vi "AutoHelper_Sequence_Execute.vi"(4 "Set Next Step":bool, 6 "Pass_Through_Time":dbl=-1.0 format="%33.4f", 8 "Use Custom Next Step":bool, 9 "Custom Step Number":T1=enum."Step 1", 10 "Initiate":bool, 11 "Step Times Sec":dbl[](array[numeric])) -> (0 "Error":bool, 1 "Elapsed Step Time":dbl, 2 "Seq  Active":bool, 3 "Step Number State":T1, 5 "New Step":bool)   [LabVIEW 2019, in "Trajectory_Library.lvlib"]
doc: "Implements a simplified state machine similar to a mechanical / electrical drum sequencer. When the Drum Sequencer is \"Ready\" and the \"Initiate\" input becomes TRUE,, the drum sequences through its set of steps from 1 to N. After each Step is executed it is followed by a wait. During the wait the Step output indicates \"Do Nothing\". The number of Steps is determined by the number of elements in the \"Step Times\" input array. Once all the steps have been executed, the Drum Sequencer cycles bac to wait for another initiate. \n\nThere is a Cancel input that interrupts the sequence, executes the Cancel Step, performs the cancel wait, and then returns to wait for an Initiate action. \n\nIf any of the Step Times, or Cancel times are negative, or there more than 32 steps, or less than 1 step an error is signaled. The drum sequencer selects the error state and stays there.\n\nInputs:\n\nOutputs:"
uses:
  Trajectory_Library.lvlib
  Enum/AutoHelperSequence_Step_Enum.ctl
  Enum/DrumSequence_State_Enum.ctl
  Util_GetTime_U32.vi
  Util_GetTime_U64.vi
  <vilib>/Utility/semaphor.llb/Obtain Semaphore Reference.vi
  Timer_Reset.vi
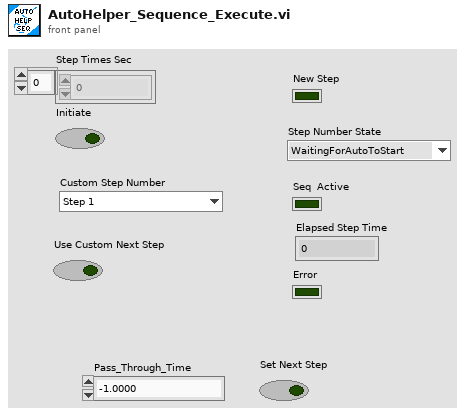
[diagram p1: front panel]
types:
  T1 = typedef "Trajectory_Library.lvlib/AutoHelperSequence_Step_Enum.ctl" = enum16{"WaitingForAutoToStart", "Step 1", "Step 2", "Step 3", "Step 4", "Step 5", "Step 6", "Step 7", "Step 8", "Step 9", "Step 10", "Step 11", "Step 12", "Step 13", "Step 14", "Step 15", "Step 16", "Step 17", "Step 18", "Step 19", "Step 20", "Step 21", "Step 22", "Step 23", "Step 24", "Step 25", "Step 26", "Step 27", "Step 28", "Step 29", "Step 30", "Step 31", "Step 32", "AutoDone"}
  T2 = typedef "Trajectory_Library.lvlib/DrumSequence_State_Enum.ctl" = enum16{"Initialize", "Ready", "First Step", "Step Wait", "Next State", "Cancel", "Cancel Wait", "Error", "Error Loop"}
  T3 = typedef "Trajectory_Library.lvlib/TIMER.ctl" = cluster{"StartTime":dbl, "Accumulated TIme":dbl, "Running":bool, "semaphore":T4}
  T4 = typedef "Semaphore RefNum" = refnum<k1>
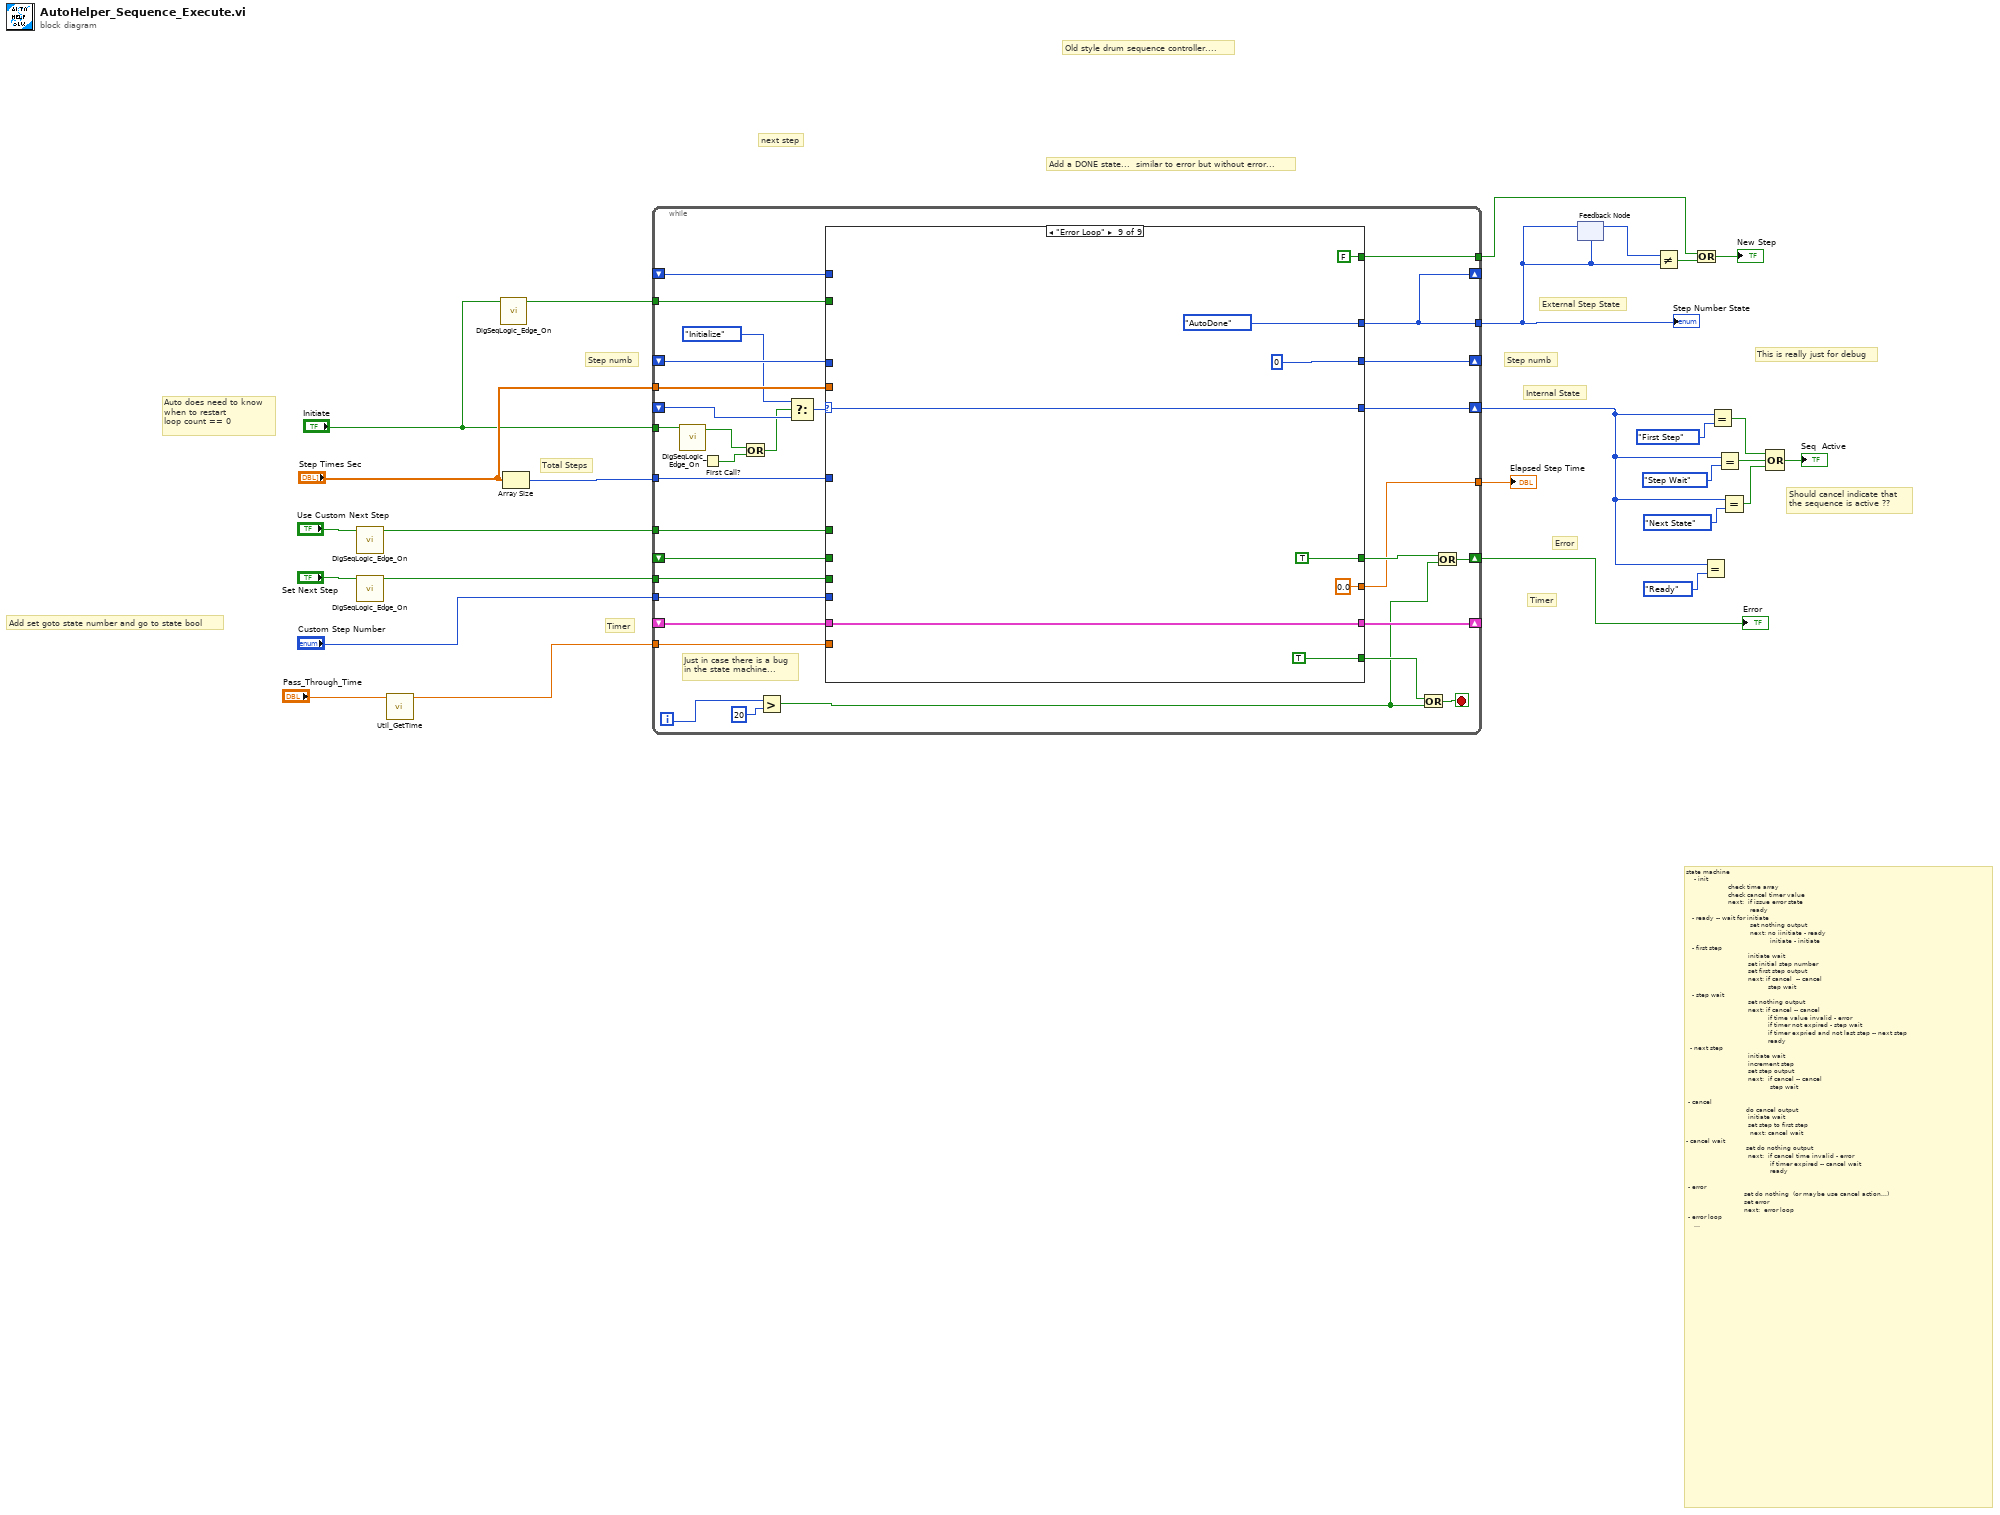
[diagram p0: block diagram]
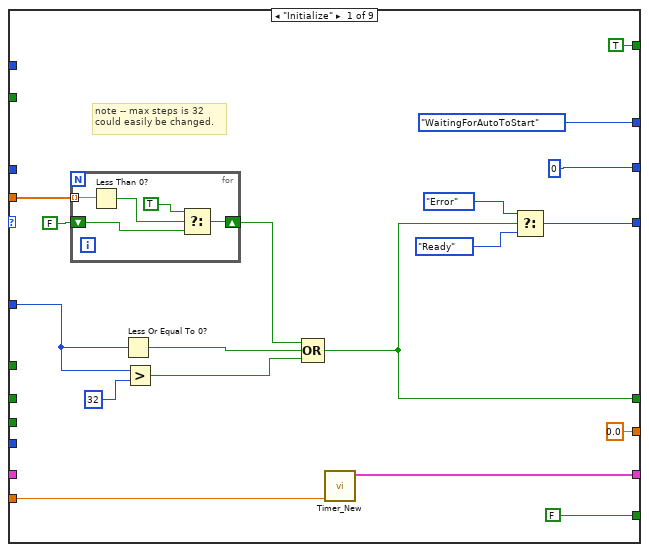
[diagram p2: hidden frame]
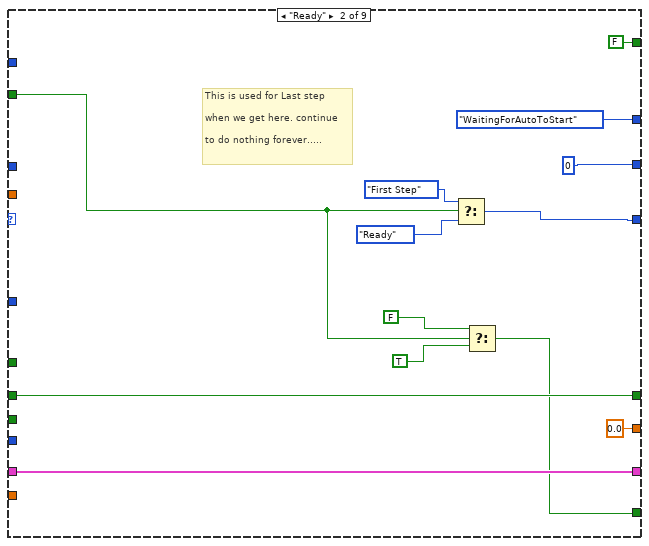
[diagram p3: hidden frame]
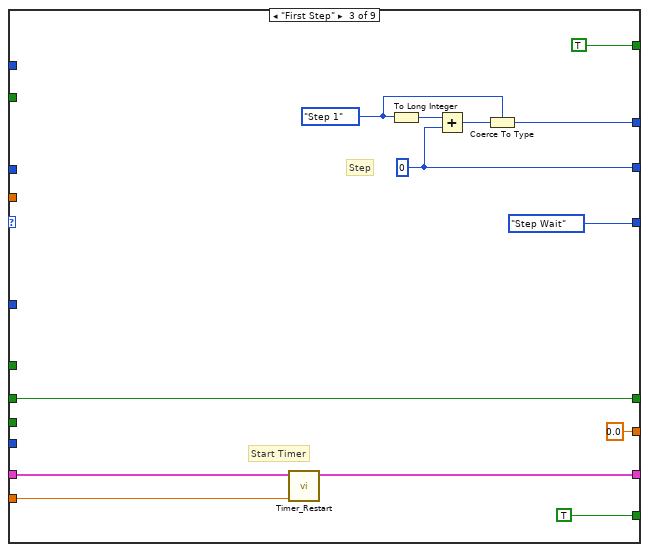
[diagram p4: hidden frame]
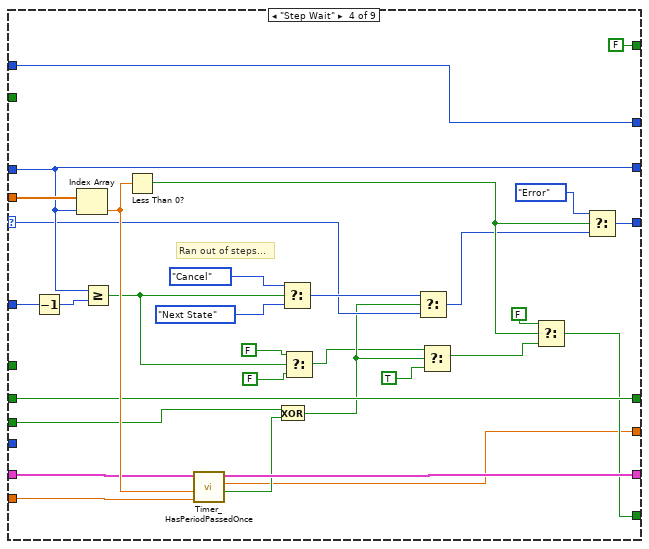
[diagram p5: hidden frame]
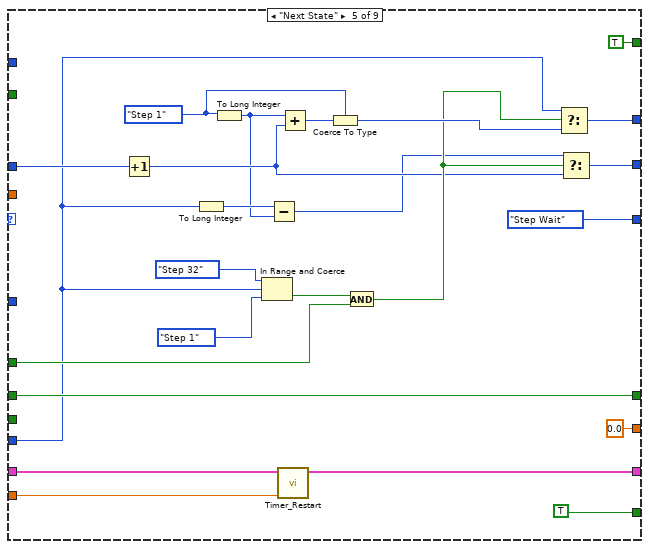
[diagram p6: hidden frame]
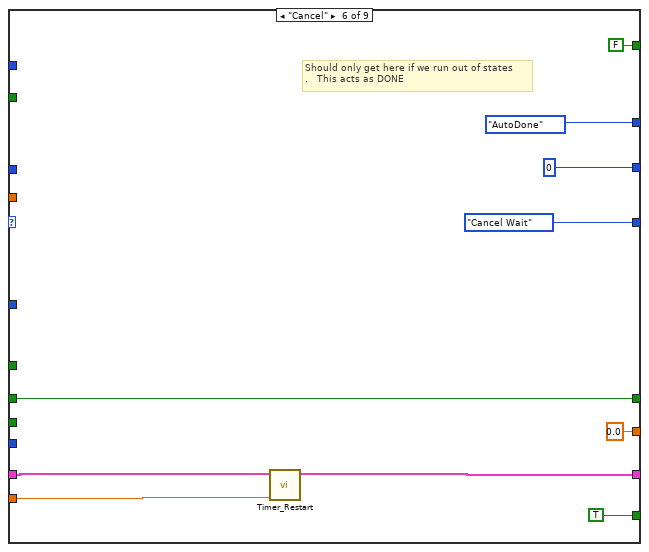
[diagram p7: hidden frame]
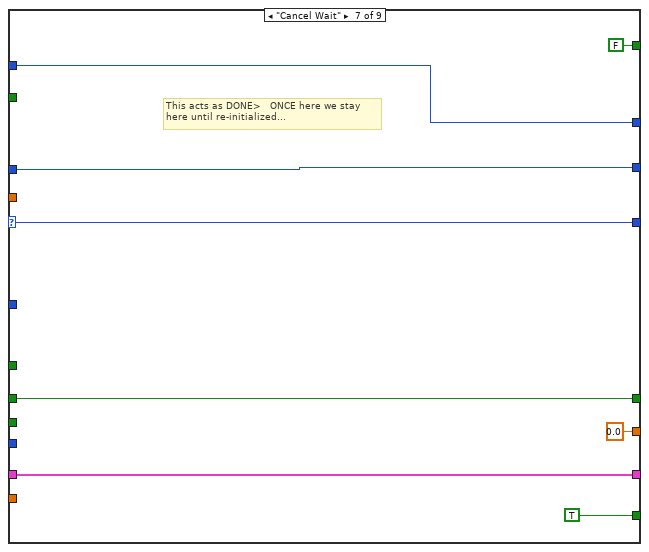
[diagram p8: hidden frame]
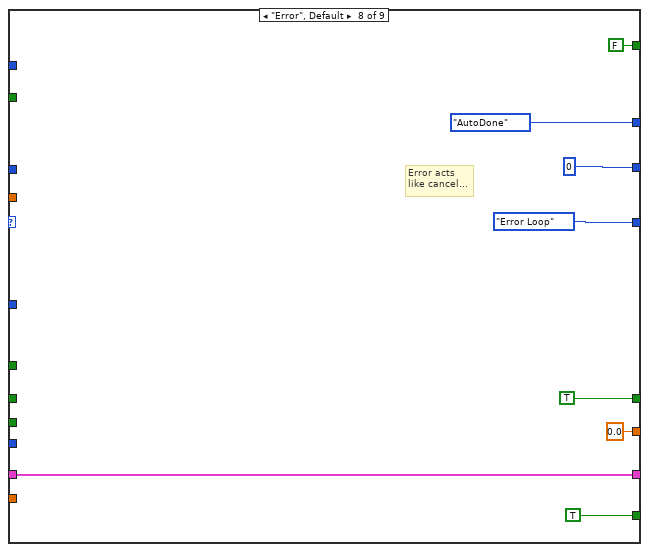
[diagram p9: hidden frame]
diagram:
  # "Add a DONE state...  similar to error but without error..."
  # "Add set goto state number and go to state bool"
  # "Auto does need to know\nwhen to restart\nloop count == 0"
  # "Should cancel indicate that\nthe sequence is active ??"
  # "This is really just for debug"
  # "Timer"
  # "Total Steps"
  # "Step numb"
  # "next step"
  # "Old style drum sequence controller...."
  # "Step numb"
  # "Timer"
  # "Error"
  # "Internal State"
  # "External Step State"
  # "state machine\n    - init\n                     check time array\n                     check cancel timer value\n                     next:  if issue error state\n                                ready\n   - ready -- wait for initiate\n                                set nothing output\n                                next: no iinitiate - ready\n                                          initiate - initiate\n   - first step \n                               initiate wait\n                               set initial step number\n                               set first step output\n                               next: if cancel  -- cancel\n                                         step wait\n   - step wait \n                               set nothing output\n                               next: if cancel -- cancel\n                                         if time value invalid - error\n                                         if timer not expired - step wait\n                                         if timer expried and not last step -- next step\n                                         ready\n  - next step\n                               initiate wait\n                               increment step\n                               set step output\n                               next:  if cancel -- cancel\n                                          step wait\n\n - cancel\n                              do cancel output\n                               initiate wait\n                               set step to first step\n                                next: cancel wait\n- cancel wait\n                              set do nothing output\n                               next:  if cancel time invalid - error\n                                          if timer expired -- cancel wait\n                                          ready\n\n - error\n                             set do nothing  (or maybe use cancel action...)\n                             set error\n                             next:  error loop\n - error loop\n                             set do nothing\n                             set error\n                             next: error loop"
  n1 = call "DigSeqLogic_Edge_On.vi"("Input"="Use Custom Next Step") -> ("On Edge"=w4:bool)  [unwired: 10 in]
  n2 = call "DigSeqLogic_Edge_On.vi"("Input"="Set Next Step") -> ("On Edge"=w13:bool)  [unwired: 10 in]
  n3 = call "Util_GetTime.vi"("Pass_Through_Time"="Pass_Through_Time") -> ("FPGA_Time_Seconds"=w24:dbl)  [unwired: 8 in, 2 out]
  n4 = call "DigSeqLogic_Edge_On.vi"("Input"="Initiate") -> ("On Edge"=w1:bool)  [unwired: 10 in]
  n5 = Array Size(array="Step Times Sec") -> (size(s)=w27:i32)
  n6 = while {
    tunnel: "Step Times Sec" -> [w57]
    tunnel: w24 -> [w56]
    tunnel: [w38] -> w8
    tunnel: w13 -> [w53]
    tunnel: w27 -> [w58]
    shift-right: [w52] -> _
    shift-left: _ -> [w46]
    shift-right: [w41] -> w12
    shift-left: _ -> [w51]
    shift-right: [w54] -> w15
    shift-left: _ -> [w48]
    shift-right: [w55] -> _
    shift-left: _ -> [w50]
    shift-right: [w38] -> _
    shift-left: _ -> [w37]
    tunnel: "Initiate" -> [w29]
    tunnel: [w34] -> w7
    tunnel: [w33] -> w6
    tunnel: w4 -> [w32]
    tunnel: "Custom Step Number" -> [w31]
    tunnel: w1 -> [w28]
    i -> [w43]
    stop <- w45 stop-if-true
    # "Just in case there is a bug\nin the state machine..."
    n7 = call "DigSeqLogic_Edge_On.vi"("Input"=w29) -> ("On Edge"=w30:bool)  [unwired: 10 in]
    n8 = First Call?() -> (First Call?: T/F=w36:bool)
    n9 = Or(x=w30, y=w36) -> (x .or. y?=w35:bool)
    n10 = Greater?(x=w43, y=20) -> (0:w39:bool)
    n11 = Select(t=DrumSequence_State_Enum."Initialize", s=w35, f=w48) -> (s? t:f=w49:T2)
    n12 = case shown="\"Error Loop\"" w49 {
      selector: w49 -> [_ _ _ w128 _ _ w174 _ w195]
      tunnel: w58 -> [w66 _ _ w126 _ _ _ _ _]
      tunnel: w57 -> [w75 _ _ w133 _ _ _ _ _]
      tunnel: [w72 w92 w99 w122 w157 w167 w179 TRUE TRUE] -> w40
      tunnel: [w69 w83 DrumSequence_State_Enum."Step Wait" w130 DrumSequence_State_Enum."Step Wait" DrumSequence_State_Enum."Cancel Wait" w174 DrumSequence_State_Enum."Error Loop" w195] -> w54
      tunnel: [w68 w91 w102 w137 w159 w170 w176 w183 w192] -> w52
      tunnel: w56 -> [w67 _ w103 w138 w160 w171 _ _ _]
      tunnel: [AutoHelperSequence_Step_Enum."WaitingForAutoToStart" ("Auto Helper Step Number") AutoHelperSequence_Step_Enum."WaitingForAutoToStart" ("Auto Helper Step Number") w105 w112 w147 AutoHelperSequence_Step_Enum."AutoDone" ("Auto Helper Step Number") w178 AutoHelperSequence_Step_Enum."AutoDone" ("Auto Helper Step Number") AutoHelperSequence_Step_Enum."AutoDone" ("Auto Helper Step Number")] -> w38
      tunnel: [0 0 w104 w129 w145 0 w180 0 0] -> w55
      tunnel: w50 -> [_ _ _ w129 w161 _ w180 _ _]
      tunnel: w53 -> [_ _ _ w124 _ _ _ _ _]
      tunnel: w46 -> [_ w91 w100 w123 w156 w165 w176 w183 w192]
      tunnel: w51 -> [_ w92 w99 w122 w157 w167 w179 _ _]
      tunnel: [FALSE w84 TRUE w113 TRUE TRUE TRUE TRUE TRUE] -> w44
      tunnel: w37 -> [_ _ _ w112 _ _ w178 _ _]
      tunnel: [TRUE FALSE TRUE FALSE TRUE FALSE FALSE FALSE FALSE] -> w34
      tunnel: [0.0 ("CurrentTImer") 0.0 ("CurrentTImer") 0.0 ("CurrentTImer") w108 0.0 ("CurrentTImer") 0.0 ("CurrentTImer") 0.0 ("CurrentTImer") 0.0 ("CurrentTImer") 0.0 ("CurrentTImer")] -> w33
      tunnel: w32 -> [_ _ _ _ w148 _ _ _ _]
      tunnel: w31 -> [_ _ _ _ w142 _ _ _ _]
      tunnel: w28 -> [_ w82 _ _ _ _ _ _ _]
      frame "Initialize" {
        # "note -- max steps is 32\ncould easily be changed."
        n13 = for {
          shift-right: [w80] -> w74
          shift-left: FALSE -> [w79]
          tunnel: w75 -> [w81] mode=indexing
          n14 = Less Than 0?(x=w81) -> (x < 0?=w77:bool)
          n15 = Select(t=TRUE, s=w77, f=w79) -> (s? t:f=w80:bool)
        }
        n16 = Less Or Equal To 0?(x=w66) -> (x <= 0?=w73:bool)
        n17 = Greater?(x=w66, y=32) -> (0:w61:bool)
        n18 = Compound Arithmetic op=OR(w74, w73, w61) -> (w72:bool)
        n19 = call "Timer_New.vi"("Pass_Through_Time"=w67) -> ("TIMER"=w68:T3)  [unwired: 10 in]
        n20 = Select(t=DrumSequence_State_Enum."Error", s=w72, f=DrumSequence_State_Enum."Ready") -> (s? t:f=w69:T2)
      }
      frame "Ready" {
        # "This is used for Last step\n\nwhen we get here. continue\n\nto do nothing forever....."
        n21 = Select(t=DrumSequence_State_Enum."First Step", s=w82, f=DrumSequence_State_Enum."Ready") -> (s? t:f=w83:T2)
        n22 = Select(t=FALSE, s=w82, f=TRUE) -> (s? t:f=w84:bool)
      }
      frame "First Step" {
        w101 = AutoHelperSequence_Step_Enum."Step 1" ("Auto Helper Step Number")
        w104 = 0
        # "Start Timer"
        # "Step"
        n23 = call "Timer_Restart.vi"("Pass_Through_Time"=w103, "in Timer"=w100) -> ("out Timer"=w102:T3)  [unwired: 9 in]
        n24 = To Long Integer(number=w101) -> (32bit integer=w107:i32)
        n25 = Add(x=w107, y=w104) -> (x+y=w106:i32)
        n26 = Coerce To Type(0:w106, 1:w101) -> (2:w105:T1)
      }
      frame "Step Wait" {
        # "Ran out of steps..."
        n27 = Decrement(x=w126) -> (x-1=w127:i32)
        n28 = Index Array(array=w133, index=w129) -> (element=w132:dbl)
        n29 = Greater Or Equal?(x=w129, y=w127) -> (x >= y?=w121:bool)
        n30 = Less Than 0?(x=w132) -> (x < 0?=w114:bool)
        n31 = call "Timer_HasPeriodPassedOnce.vi"("Pass_Through_Time"=w138, "Period"=w132, "in Timer"=w123) -> ("Expired"=w125:bool, "CurrentTImer"=w108:dbl, "out Timer"=w137:T3)  [unwired: 6 in]
        n32 = Exclusive Or(1:w125, 2:w124) -> (0:w118:bool)
        n33 = Select(t=DrumSequence_State_Enum."Cancel", s=w121, f=DrumSequence_State_Enum."Next State") -> (s? t:f=w134:T2)
        n34 = Select(t=FALSE, s=w121, f=FALSE) -> (s? t:f=w117:bool)
        n35 = Select(t=w134, s=w118, f=w128) -> (s? t:f=w111:T2)
        n36 = Select(t=w117, s=w118, f=TRUE) -> (s? t:f=w110:bool)
        n37 = Select(t=FALSE, s=w114, f=w110) -> (s? t:f=w113:bool)
        n38 = Select(t=DrumSequence_State_Enum."Error", s=w114, f=w111) -> (s? t:f=w130:T2)
      }
      frame "Next State" {
        w158 = AutoHelperSequence_Step_Enum."Step 1" ("Auto Helper Step Number")
        n39 = Increment(x=w161) -> (x+1=w143:i32)
        n40 = To Long Integer(number=w142) -> (32bit integer=w141:i32)
        n41 = To Long Integer(number=w158) -> (32bit integer=w140:i32)
        n42 = In Range and Coerce(upper limit=AutoHelperSequence_Step_Enum."Step 32" ("Auto Helper Step Number"), x=w142, lower limit=AutoHelperSequence_Step_Enum."Step 1" ("Auto Helper Step Number")) -> (In Range?=w149:bool)  [unwired: 1 out]
        n43 = Subtract(x=w141, y=w140) -> (x-y=w139:i32)
        n44 = call "Timer_Restart.vi"("Pass_Through_Time"=w160, "in Timer"=w156) -> ("out Timer"=w159:T3)  [unwired: 9 in]
        n45 = Add(x=w140, y=w143) -> (x+y=w162:i32)
        n46 = Coerce To Type(0:w162, 1:w158) -> (2:w146:T1)
        n47 = And(x=w149, y=w148) -> (x .and. y?=w144:bool)
        n48 = Select(t=w142, s=w144, f=w146) -> (s? t:f=w147:T1)
        n49 = Select(t=w139, s=w144, f=w143) -> (s? t:f=w145:i32)
      }
      frame "Cancel" {
        # "Should only get here if we run out of states\n.   This acts as DONE"
        n50 = call "Timer_Restart.vi"("Pass_Through_Time"=w171, "in Timer"=w165) -> ("out Timer"=w170:T3)  [unwired: 9 in]
      }
      frame "Cancel Wait" {
        # "This acts as DONE>   ONCE here we stay \nhere until re-initialized..."
      }
      frame "Error", Default {
        # "Error acts\nlike cancel..."
      }
      frame "Error Loop" {
      }
    }
    n51 = Or(x=w44, y=w39) -> (x .or. y?=w45:bool)
    n52 = Or(x=w40, y=w39) -> (x .or. y?=w41:bool)
  }
  "Error" <- w12
  "Step Number State" <- w8
  "Elapsed Step Time" <- w6
  n53 = feedback #1(w8) -> (w11:T1)
  n54 = feedback-in #1(w8) -> ()
  n55 = Not Equal?(x=w11, y=w8) -> (x != y?=w9:bool)
  n56 = Or(x=w7, y=w9) -> (x .or. y?=→"New Step":bool)
  n57 = Equal?(x=w15, y=DrumSequence_State_Enum."Ready") -> ()  [unwired: 1 out]
  n58 = Equal?(x=w15, y=DrumSequence_State_Enum."First Step") -> (x = y?=w19:bool)
  n59 = Equal?(x=w15, y=DrumSequence_State_Enum."Step Wait") -> (x = y?=w18:bool)
  n60 = Equal?(x=w15, y=DrumSequence_State_Enum."Next State") -> (x = y?=w17:bool)
  n61 = Compound Arithmetic op=OR(w19, w18, w17) -> (→"Seq  Active":bool)
